vi "getSettingDirectory.vi"(11 "BaseSetting in":refnum<class "Setting.lvclass">) -> (2 "SettingDirectory":path, 3 "BaseSetting out":refnum<class "Setting.lvclass">)   [LabVIEW 2016, in "Settings.lvlib" / "Setting.lvclass"]
uses:
  Setting.lvclass
  Setting.lvclass/Setting.ctl
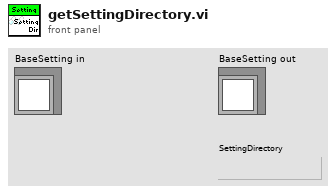
[diagram p1: front panel]
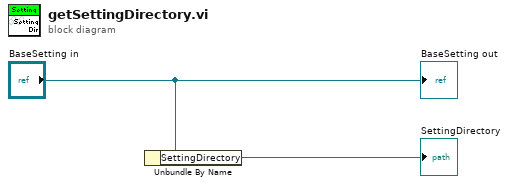
[diagram p0: block diagram]
diagram:
  n1 = Unbundle By Name("BaseSetting in") -> ("SettingDirectory"=→"SettingDirectory":path)
  "BaseSetting out" <- "BaseSetting in"
